vi "add PID to engine.vi"(8 "error in (no error)":errorcluster, 9 "line item in":T1, 10 "engine configuration":refnum<class "engine configuration.lvclass">, 11 "Tagbus PID Module configuration in":refnum<class "Tagbus PID Module configuration.lvclass">) -> (0 "error out":errorcluster, 2 "engine configuration out":refnum<class "engine configuration.lvclass">, 3 "Tagbus PID Module configuration out":refnum<class "Tagbus PID Module configuration.lvclass">)   [LabVIEW 2014, in "Tagbus PID Module editor node.lvclass"]
uses:
  Tagbus PID Module editor node.lvclass
  <vilib>/NI/Module Execution Interface/Engine Configuration/engine configuration.lvclass
  module/configuration/Tagbus PID Module configuration.lvclass
  PID array element.ctl
  <vilib>/NI/Configuration Framework/serializable configuration/NISE_CEF_serializable configuration.lvclass/NISE_CEF_serializable configuration.ctl
  <vilib>/Utility/LVClass/Get LV Class Name.vi
  <vilib>/NI/Configuration Framework/error generator/NISE_error generator.vi
  <vilib>/NI/Configuration Framework/serializable configuration/NISE_CEF_serializable configuration.lvclass
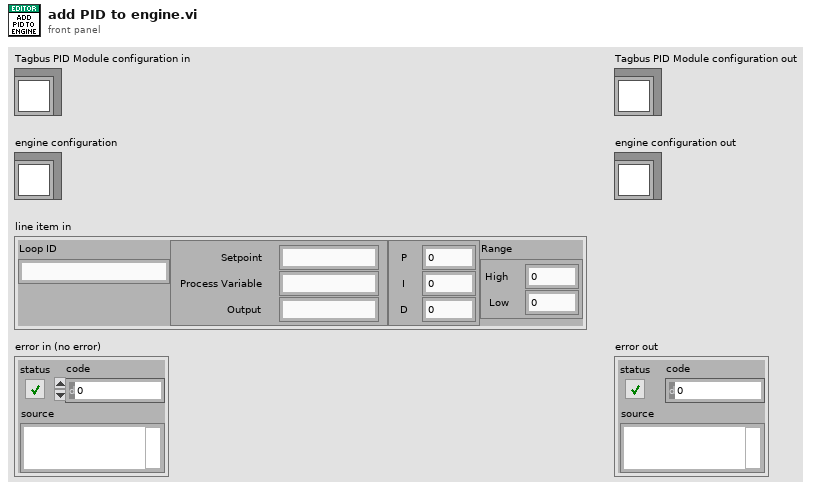
[diagram p1: front panel]
types:
  T1 = typedef "Tagbus PID Module editor node.lvclass/PID array element.ctl" = cluster{"Loop ID":string, "Tags":cluster{"Setpoint":string, "Process Variable":string, "Output":string}, "Gains":cluster{"P":dbl, "I":dbl, "D":dbl}, "Range":cluster{"High":dbl, "Low":dbl}}
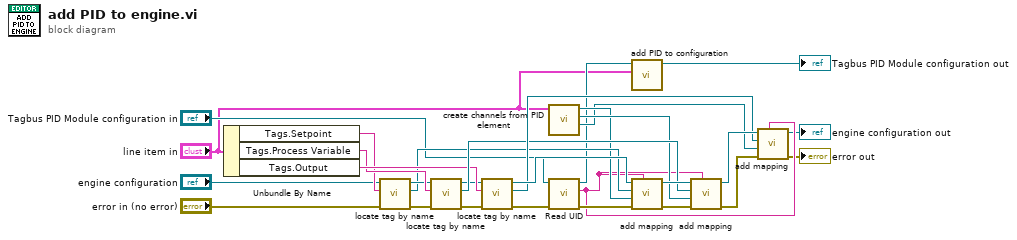
[diagram p0: block diagram]
diagram:
  n1 = Unbundle By Name("line item in") -> ("Tags.Setpoint"=w12:string, "Tags.Process Variable"=w15:string, "Tags.Output"=w17:string)
  n2 = call <vilib>:"locate tag by name.vi"("error in"="error in (no error)", "tag name"=w12, "engine configuration in"="engine configuration") -> ("error out"=w19:errorcluster, "tag descriptor"=w13:refnum<class "tag descriptor.lvclass">, "engine configuration out"=w14:refnum<class "engine configuration.lvclass">)  [unwired: 6 in]
  n3 = call <vilib>:"locate tag by name.vi"("error in"=w19, "tag name"=w15, "engine configuration in"=w14) -> ("error out"=w18:errorcluster, "tag descriptor"=w20:refnum<class "tag descriptor.lvclass">, "engine configuration out"=w16:refnum<class "engine configuration.lvclass">)  [unwired: 6 in]
  n4 = call <vilib>:"locate tag by name.vi"("error in"=w18, "tag name"=w17, "engine configuration in"=w16) -> ("error out"=w26:errorcluster, "tag descriptor"=w21:refnum<class "tag descriptor.lvclass">, "engine configuration out"=w27:refnum<class "engine configuration.lvclass">)  [unwired: 6 in]
  n5 = call "create channels from PID element.vi"("line item in"="line item in") -> ("channel 3"=w8:refnum<class "TBM channel.lvclass">, "channel"=w10:refnum<class "TBM channel.lvclass">, "TBM channel out"=w9:refnum<class "TBM channel.lvclass">)  [unwired: 8 in]
  n6 = call <vilib>:"Read UID.vi"("error in"=w26, "configuration in"="Tagbus PID Module configuration in") -> ("error out"=w22:errorcluster, "instance id"=w7:string, "configuration out"=w3:refnum<class "Tagbus PID Module configuration.lvclass">)  [unwired: 7 in]
  n7 = call "add PID to configuration.vi"("PID Element in"="line item in", "Tagbus PID Module configuration in"=w3) -> ("Tagbus PID Module configuration out"=→"Tagbus PID Module configuration out":refnum<class "Tagbus PID Module configuration.lvclass">)  [unwired: 8 in, 1 out]
  n8 = call <vilib>:"add mapping.vi"("owner ID"=w7, "error in"=w22, "channel"=w9, "tag descriptor"=w13, "engine configuration"=w27) -> ("error out"=w23:errorcluster, "engine configuration out"=w28:refnum<class "engine configuration.lvclass">)  [unwired: 5 in]
  n9 = call <vilib>:"add mapping.vi"("owner ID"=w7, "error in"=w23, "channel"=w10, "tag descriptor"=w20, "engine configuration"=w28) -> ("error out"=w24:errorcluster, "engine configuration out"=w29:refnum<class "engine configuration.lvclass">)  [unwired: 5 in]
  n10 = call <vilib>:"add mapping.vi"("owner ID"=w7, "error in"=w24, "channel"=w8, "tag descriptor"=w21, "engine configuration"=w29) -> ("error out"=→"error out":errorcluster, "engine configuration out"=→"engine configuration out":refnum<class "engine configuration.lvclass">)  [unwired: 5 in]
